vi "Scope Get Trace State Machine.vi"(7 "Type Measurement":string="LSV", 8 "error in (no error)":errorcluster, 10 "Data Queue":refnum<queue>, 11 "Queue in":refnum<queue>) -> (0 "error out":errorcluster, 2 "Measurements":dbl[](array[numeric]), 3 "Results":T1)   [LabVIEW 2020]
uses:
  <instrlib>/PalmSens SDK for LabVIEW 5.10/PalmSens/MeasurementResults.ctl
  <instrlib>/PalmSens SDK for LabVIEW 5.10/PalmSens/LiveCurveResult.ctl
  Message Queue/Message Cluster.ctl
  PCT FGV CMD.ctl
  Message Queue/Message Queue.lvlib
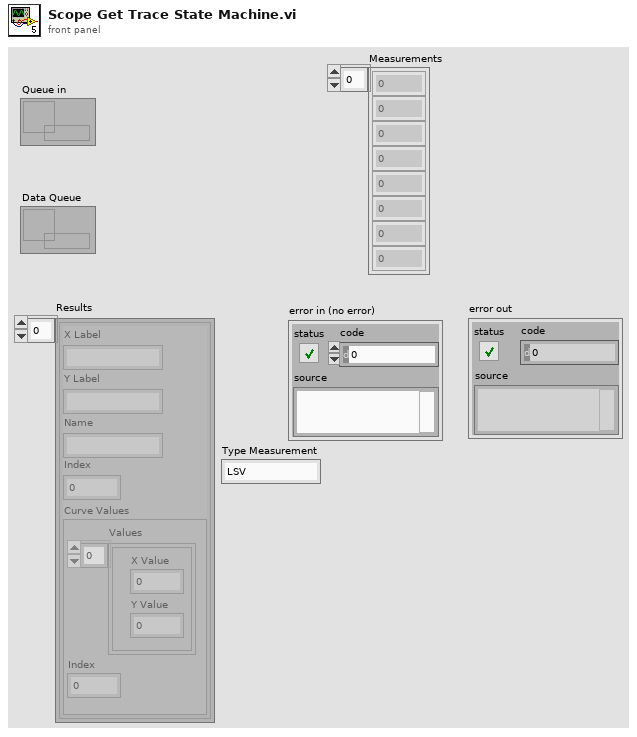
[diagram p1: front panel]
types:
  T1 = typedef "MeasurementResults.ctl" = T2[]
  T2 = typedef "LiveCurveResult.ctl" = cluster{"X Label":string, "Y Label":string, "Name":string, "Index":i16, "Curve Values":cluster{"Values":cluster{"X Value":dbl, "Y Value":dbl}[], "Index":i16}}
  T3 = cluster{"Next Step":string, "Trigger Level":dbl, "Timebase":dbl, "Source (0: Channel 1) 2":u16[]}
  T4 = cluster{"Next Step":string, "Trigger Level":dbl, "Timebase":dbl, "Source (0: Channel 1)":u16[]}
  T5 = typedef "PCT FGV CMD.ctl" = enum16{"INIT", "GET", "SET"}
  T6 = cluster{"Type CMD":string, "Mode CMD":string, "Main CMD":string}
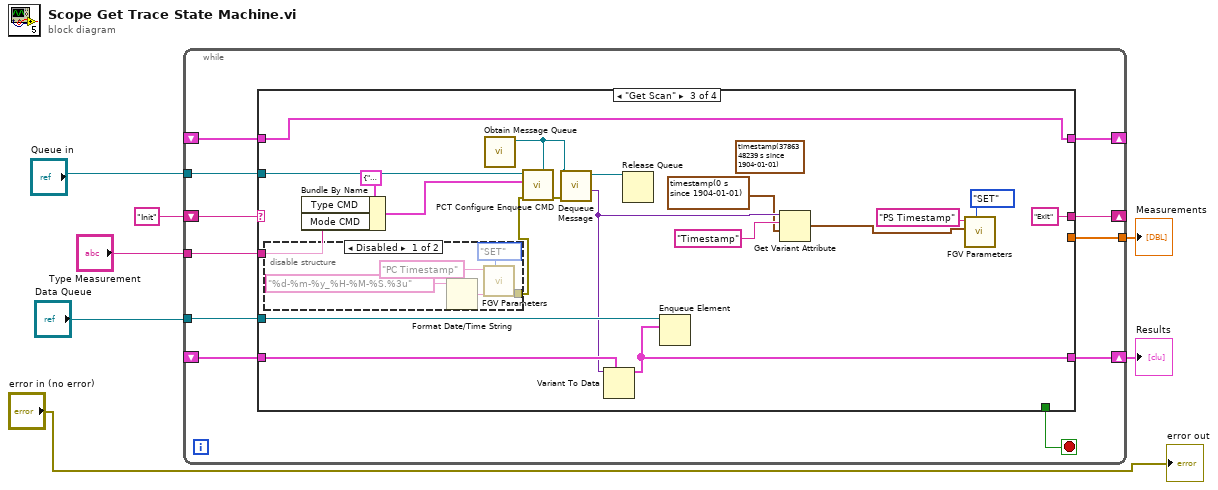
[diagram p0: block diagram]
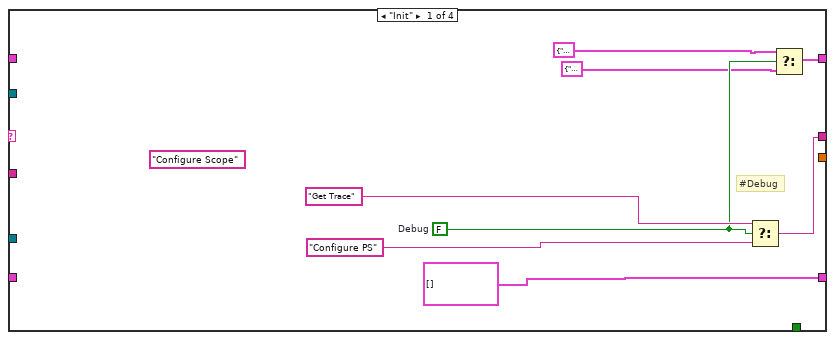
[diagram p2: hidden frame]
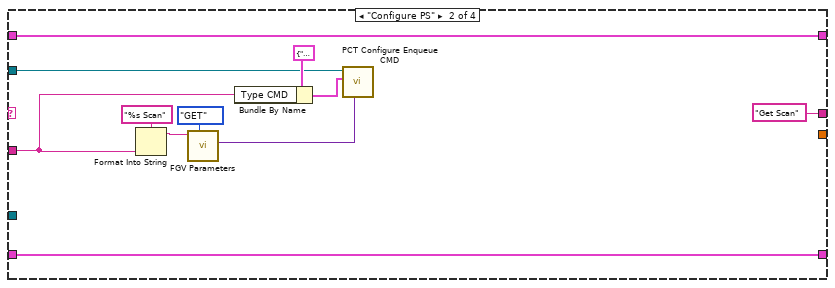
[diagram p3: hidden frame]
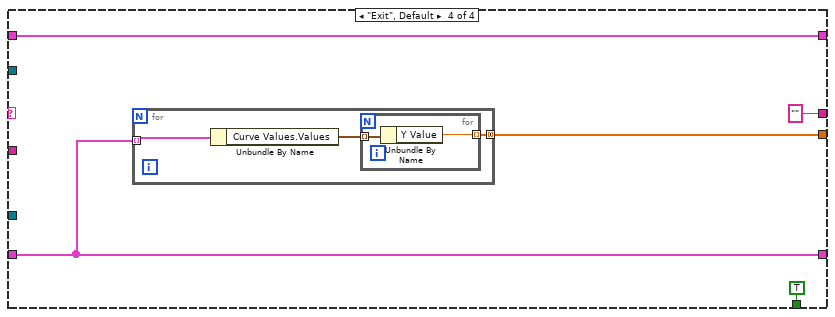
[diagram p5: hidden frame]
diagram:
  n1 = while {
    shift-right: [w17] -> _
    shift-left: "Init" -> [w18]
    shift-right: [w16] -> _
    shift-left: _ -> [w15]
    tunnel: "Queue in" -> [w14]
    tunnel: "Data Queue" -> [w12]
    shift-right: [w11] -> w4
    shift-left: _ -> [w10]
    tunnel: [w9] -> w3
    tunnel: "Type Measurement" -> [w8]
    stop <- w13 stop-if-true
    n2 = case shown="\"Get Scan\"" w18 {
      tunnel: [w24 "Get Scan" "Exit" ("Next Step") "" ("Next Step")] -> w17
      tunnel: [w20 w37 w55 w64] -> w16
      tunnel: w15 -> [_ w37 w55 w64]
      tunnel: w14 -> [_ w33 w56 _]
      tunnel: [_ _ _ TRUE] -> w13
      tunnel: w12 -> [_ _ w54 _]
      tunnel: [T1 [] ("Results") w35 w47 w63] -> w11
      tunnel: w10 -> [_ w35 w49 w63]
      tunnel: [_ _ _ w62] -> w9
      tunnel: w8 -> [_ w29 w45 _]
      frame "Init" {
        w23 = FALSE  # Debug
        (unwired) "Configure Scope"
        # "#Debug"
        n3 = Select(t="Get Trace", s=w23, f="Configure PS") -> (s? t:f=w24:string)
        n4 = Select(t=T4 {"Next Step"="Exit", "Trigger Level"=2.0, "Timebase"=0.1, "Source (0: Channel 1)"=[0, 1, 2]}, s=w23, f=T3 {"Next Step"="Configure Scope", "Trigger Level"=2.0, "Timebase"=0.1, "Source (0: Channel 1) 2"=[0, 1, 2]}) -> (s? t:f=w20:T3)
      }
      frame "Configure PS" {
        n5 = Format Into String(format string="%s Scan" ("Key"), w29) -> (resulting string=w28:string)  [unwired: 2 in, 1 out]
        n6 = call "FGV Parameters.vi"("CMD"=PCT_FGV_CMD."GET", "Key"=w28) -> ("output"=w31:variant)  [unwired: 7 in, 2 out]
        n7 = Bundle By Name(cluster=T6 {"Type CMD"="LSV", "Mode CMD"="", "Main CMD"="Configure"} ("CMD"), "Type CMD"=w29) -> (w32:T6)
        n8 = call "PCT Configure Enqueue CMD.vi"("Parameter Data"=w31, "CMD"=w32, "CMD Queue in"=w33) -> ()  [unwired: 6 in, 3 out]
      }
      frame "Get Scan" {
        (unwired) timestamp(3786348239.585165 s since 1904-01-01) ("TimeStamp 2")
        n9 = disable-structure shown="Disabled" {
          disable-tunnel: [w57 _] -> w38
          frame Disabled {
            n10 = Format Date/Time String(time format string (%c)="%d-%m-%y_%H-%M-%S.%3u") -> (date/time string=w58:string)  [unwired: 2 in]
            n11 = call "FGV Parameters.vi"("CMD"=PCT_FGV_CMD."SET", "input"=w58, "Key"="PC Timestamp") -> ("error out"=w57:errorcluster)  [unwired: 6 in, 2 out]
          }
          frame Enabled {
          }
        }
        n12 = Bundle By Name(cluster=T6 {"Type CMD"="LSV", "Mode CMD"="LSV", "Main CMD"="Data"} ("CMD"), "Type CMD"=w45, "Mode CMD"=w45) -> (w46:T6)
        n13 = call "Obtain Message Queue.vi"() -> ("Message Queue"=w53:refnum<queue>)  [unwired: 10 in, 1 out]
        n14 = call "PCT Configure Enqueue CMD.vi"("Response Queue"=w53, "error in (no error)"=w38, "CMD"=w46, "CMD Queue in"=w56) -> ("error out"=w52:errorcluster)  [unwired: 5 in, 2 out]
        n15 = call "Dequeue Message.vi"("error in (no error)"=w52, "Message Queue"=w53) -> ("Message Data"=w44:variant, "dup Message Queue"=w51:refnum<queue>)  [unwired: 6 in, 2 out]
        n16 = Variant To Data(type=w49, Variant=w44) -> (data=w47:T1)  [unwired: 1 in, 1 out]
        n17 = Release Queue(queue=w51) -> ()  [unwired: 2 in, 3 out]
        n18 = Enqueue Element(queue=w54, element=w47) -> ()  [unwired: 2 in, 3 out]
        n19 = Get Variant Attribute(Variant=w44, name="Timestamp", default value (empty Variant)=timestamp(0 s since 1904-01-01) ("TimeStamp 2")) -> (value=w39:timestamp)  [unwired: 1 in, 3 out]
        n20 = call "FGV Parameters.vi"("CMD"=PCT_FGV_CMD."SET", "input"=w39, "Key"="PS Timestamp") -> ()  [unwired: 6 in, 3 out]
      }
      frame "Exit", Default {
        n21 = for {
          tunnel: w63 -> [w69] mode=indexing
          tunnel: [w67] -> w62 mode=concatenating
          n22 = Unbundle By Name(w69) -> ("Curve Values.Values"=w68:cluster{"X Value":dbl, "Y Value":dbl}[])
          n23 = for {
            tunnel: w68 -> [w71] mode=indexing
            tunnel: [w70] -> w67 mode=indexing
            n24 = Unbundle By Name(w71) -> ("Y Value"=w70:dbl)
          }
        }
      }
    }
  }
  "Results" <- w4
  "Measurements" <- w3
  "error out" <- "error in (no error)"
